vi "Abrir_central_todos_certificados.vi"() -> ()   [LabVIEW 2019]
uses:
  <vilib>/Utility/config.llb/Config Data RefNum.ctl
  <vilib>/Utility/config.llb/Write Key (Path).vi
  <vilib>/Utility/config.llb/NI_LVConfig.lvlib
panel:
  in  "Search Button":bool
  in  "barra_de_pesquisa":string
  in  "Editor Vinculos":bool
  in  "Stop Button":bool
  in  "Array":T1(array[cluster])
  out "Array Tags":string[](array[string])
  out "Section Names":string[](array[string])
  out "refnum out":T2
  out "error out":errorcluster
  # "Digite no campo de busca a TAG desejada:"
  # "Digite no campo de busca a TAG desejada:"
  # "SELECIONE A TAG A QUAL\nDESEJA ABRIR O PDF COM \nO CERTIFICADO DE CALIBRA敲O"
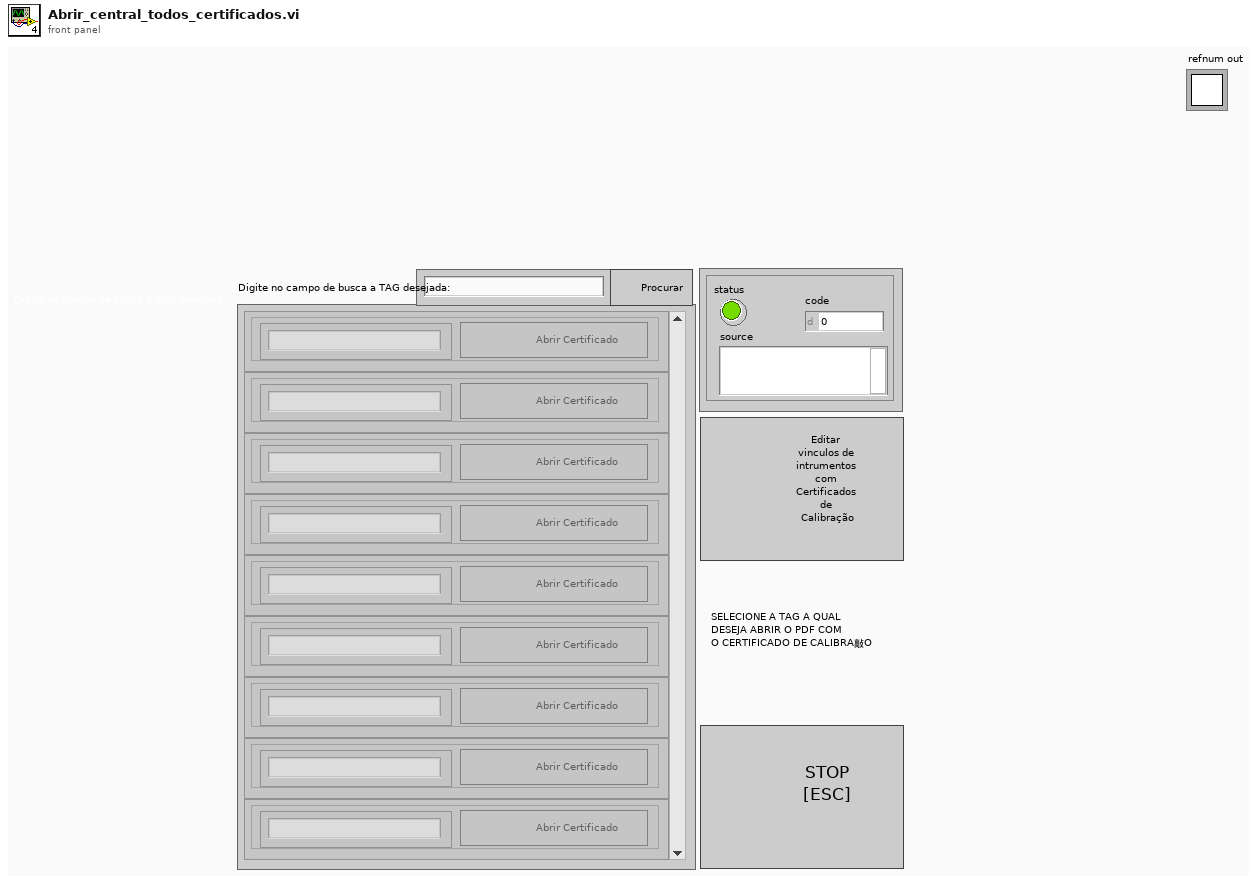
[diagram p1: front panel]
types:
  T1 = cluster{"TAG":string, "Abrir Certificado":bool}[]
  T2 = typedef "NI_LVConfig.lvlib/Config Data RefNum.ctl" = refnum<k1>
  T3 = enum8{"Enabled", "Disabled", "Disabled and Grayed Out"}
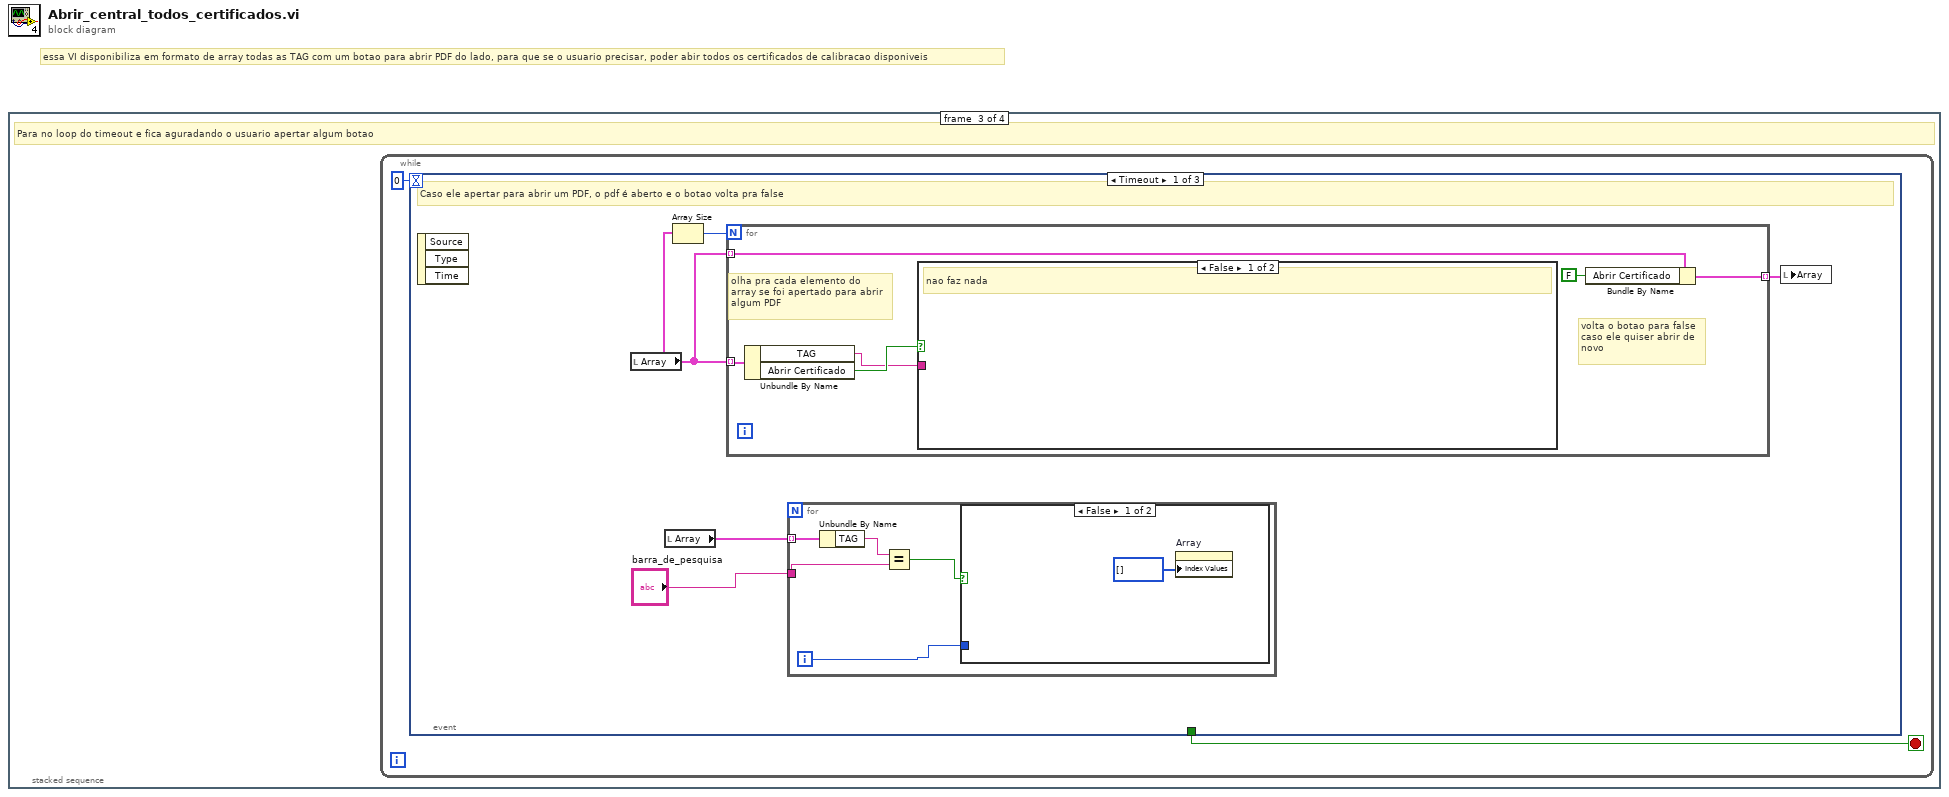
[diagram p0: block diagram]
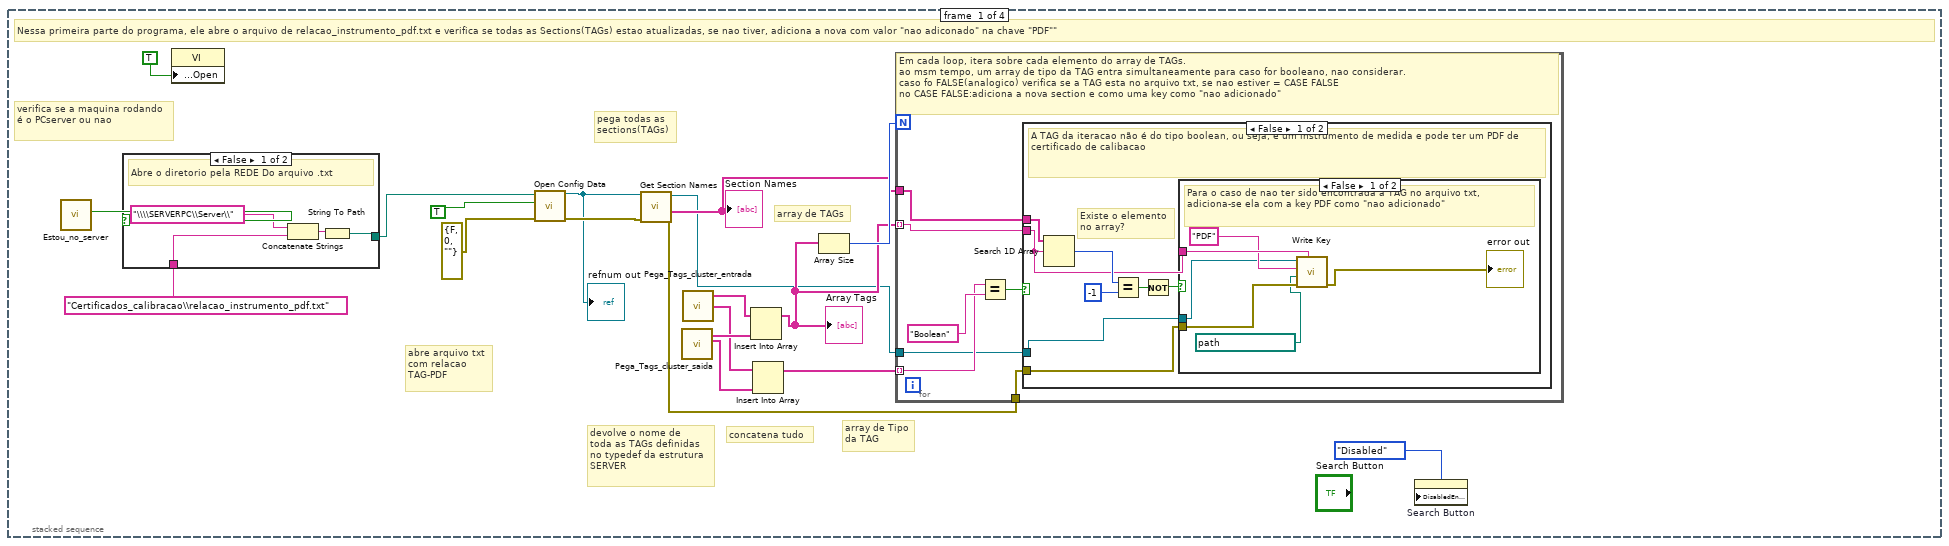
[diagram p2: hidden frame]
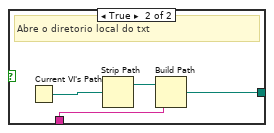
[diagram p3: hidden frame]
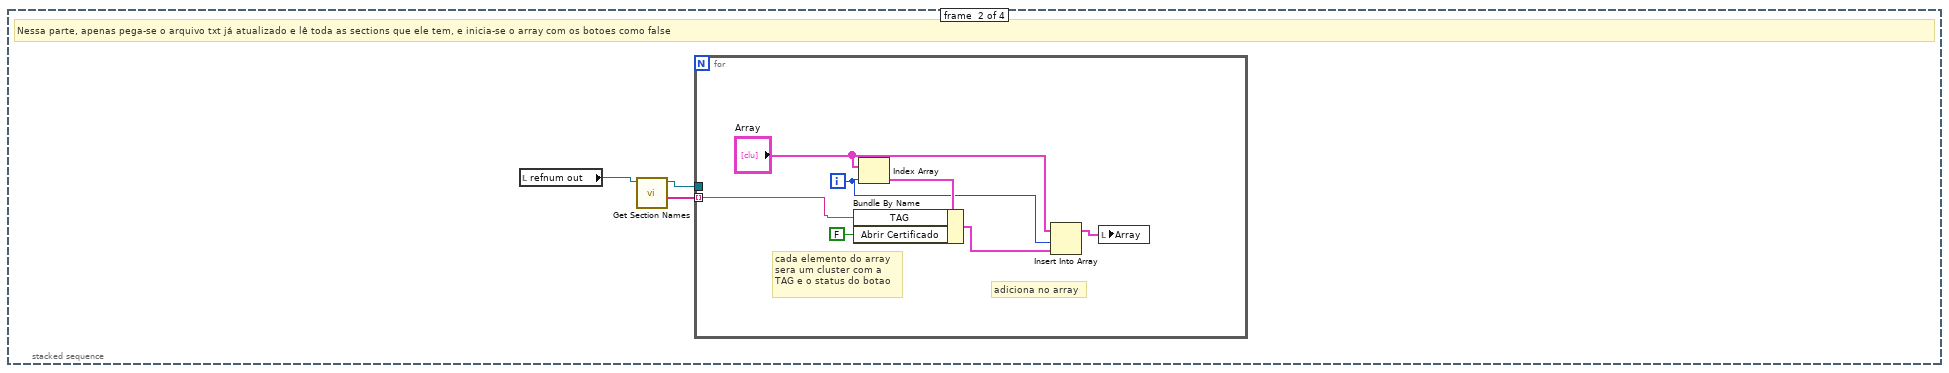
[diagram p6: hidden frame]
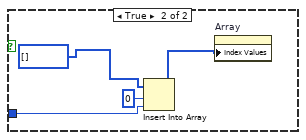
[diagram p7: hidden frame]
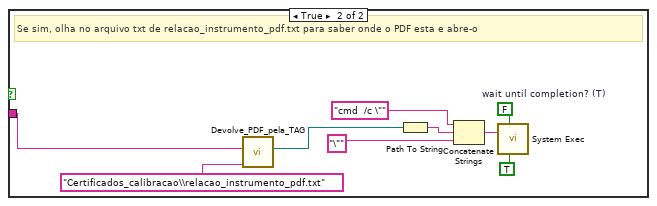
[diagram p8: hidden frame]
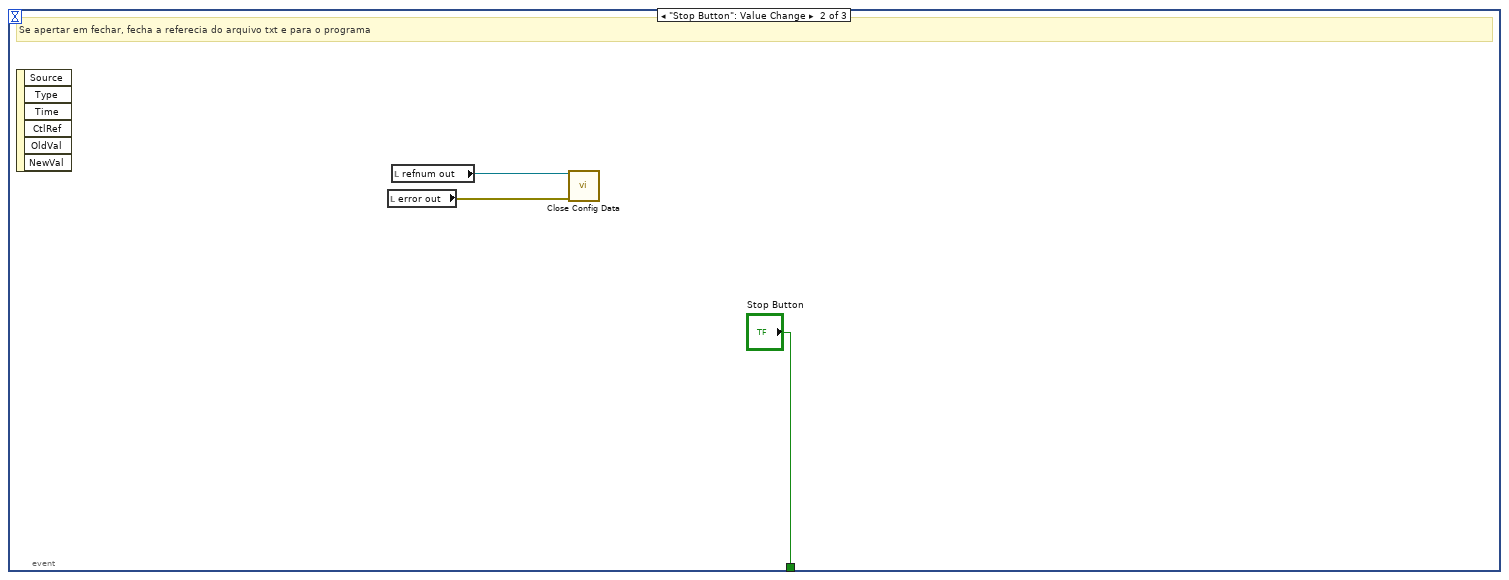
[diagram p9: hidden frame]
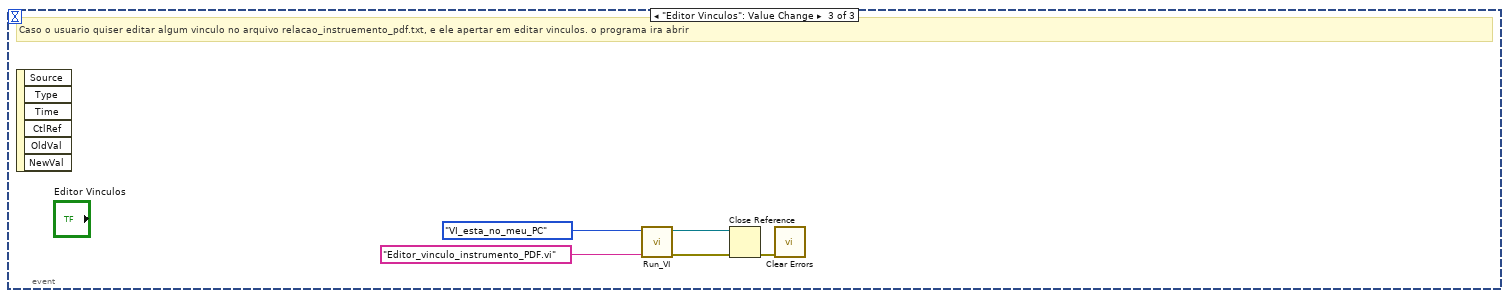
[diagram p10: hidden frame]
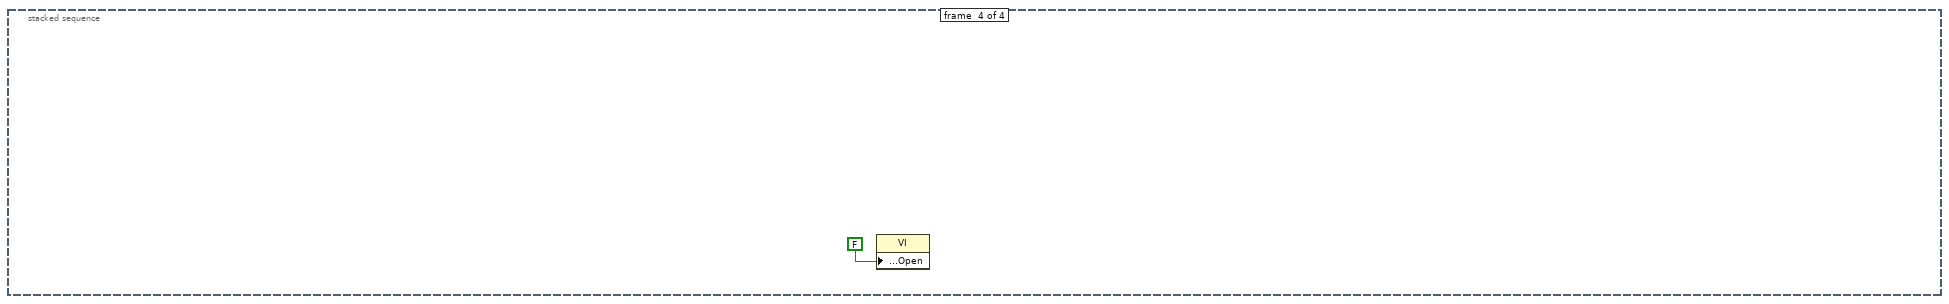
[diagram p11: hidden frame]
diagram:
  # "essa VI disponibiliza em formato de array todas as TAG com um botao para abrir PDF do lado, para que se o usuario precisar, poder abir todos os certificados de calibracao disponiveis"
  n1 = stacked-sequence {
    frame #0 {
      # "array de TAGs"
      # "array de Tipo\nda TAG"
      # "concatena tudo"
      # "devolve o nome de\ntoda as TAGs definidas\nno typedef da estrutura\nSERVER"
      # "pega todas as\nsections(TAGs)"
      # "abre arquivo txt\ncom relacao\nTAG-PDF"
      # "verifica se a maquina rodando é o PCserver ou nao"
      # "Nessa primeira parte do programa, ele abre o arquivo de relacao_instrumento_pdf.txt e verifica se todas as Sections(TAGs) estao atualizadas, se nao tiver, adiciona a nova com valor \"nao adiconado\" na chave \"PDF\"\""
      n2 = call "Estou_no_server.vi"() -> ("Estou no serve?"=w3:bool)  [unwired: 11 in]
      n3 = case shown="False" w3 {
        tunnel: [w21 w26] -> w2
        tunnel: "Certificados_calibracao\\relacao_instrumento_pdf.txt" ("name or relative path") -> [w22 w25]
        frame False {
          # "Abre o diretorio pela REDE Do arquivo .txt"
          n4 = Concatenate Strings("\\\\SERVERPC\\Server\\", w22) -> (w20:string)
          n5 = String To Path(string=w20) -> (path=w21:path)
        }
        frame True {
          # "Abre o diretorio local do txt"
          n6 = Current VI's Path() -> (path=w24:path)
          n7 = Strip Path(path=w24) -> (stripped path=w27:path)  [unwired: 1 out]
          n8 = Build Path(base path=w27, name or relative path=w25) -> (appended path=w26:path)
        }
      }
      n9 = property class="VI"("Front Panel.Open"=TRUE ("Front Panel Window:Open")) -> ()  [unwired: 2 in, 2 out]
      n10 = call <vilib>:"Open Config Data.vi"("error in (no error)"=errorcluster {"status"=FALSE, "code"=0, "source"=""}, "create file if necessary (T)"=TRUE, "configuration file path"=w2) -> ("error out"=w16:errorcluster, "refnum"=w15:T2)  [unwired: 6 in, 1 out]
      "refnum out" <- w15
      n11 = call <vilib>:"Get Section Names.vi"("error in (no error)"=w16, "refnum"=w15) -> ("error out"=w5:errorcluster, "section names"=w11:string[], "refnum out"=w6:T2)  [unwired: 7 in]
      "Section Names" <- w11
      n12 = call "Pega_Tags_cluster_saida.vi"() -> ("TipoTag"=w8:string[], "Array Tags"=w13:string[])  [unwired: 10 in]
      n13 = call "Pega_Tags_cluster_entrada.vi"() -> ("TipoVariavel"=w9:string[], "Array Tags"=w14:string[])  [unwired: 4 in]
      n14 = Insert Into Array(array=w14, new element=w13) -> (w10:string[])  [unwired: 1 in]
      "Array Tags" <- w10
      n15 = Insert Into Array(array=w9, new element=w8) -> (w7:string[])  [unwired: 1 in]
      n16 = Array Size(array=w10) -> (size(s)=w12:i32)
      n17 = for {
        N: w12 -> [_]
        tunnel: w10 -> [w31] mode=indexing
        tunnel: w11 -> [w30]
        tunnel: w7 -> [w33] mode=indexing
        tunnel: w6 -> [w29]
        tunnel: w5 -> [w28]
        # "Em cada loop, itera sobre cada elemento do array de TAGs.\nao msm tempo, um array de tipo da TAG entra simultaneamente para caso for booleano, nao considerar.\ncaso fo FALSE(analogico) verifica se a TAG esta no arquivo txt, se nao estiver = CASE FALSE\nno CASE FALSE:adiciona a nova section e como uma key como \"nao adicionado\""
        n18 = Equal?(x=w33, y="Boolean") -> (x = y?=w32:bool)
        n19 = case shown="False" w32 {
          tunnel: w31 -> [w37 _]
          tunnel: w30 -> [w40 _]
          tunnel: w29 -> [w36 _]
          tunnel: w28 -> [w35 _]
          frame False {
            # "Existe o elemento\nno array?"
            # "A TAG da iteracao não é do tipo boolean, ou seja, é um instrumento de medida e pode ter um PDF de certificado de calibacao"
            n20 = Search 1D Array(1D array=w40, element=w37) -> (index of element=w39:i32)  [unwired: 1 in]
            n21 = Equal?(x=w39, y=-1) -> (x = y?=w42:bool)
            n22 = Not(x=w42) -> (.not. x?=w38:bool)
            n23 = case shown="False" w38 {
              tunnel: w37 -> [w48 _]
              tunnel: w36 -> [w46 _]
              tunnel: w35 -> [w45 _]
              frame False {
                # "Para o caso de nao ter sido encontrada a TAG no arquivo txt,\nadiciona-se ela com a key PDF como \"nao adicionado\""
                n24 = call-poly <vilib>:"Write Key.vi"("section"=w48, "error in (no error)"=w45, "value"=path "Não Adicionado", "key"="PDF", "refnum"=w46) -> ("error out"=→"error out":errorcluster)  [unwired: 4 in, 2 out]
              }
              frame True {
              }
            }
          }
          frame True {
            # "a TAG analisada é uma booleana"
          }
        }
      }
      n25 = property on="Search Button" class="Bool"("DisabledEnum"=T3."Disabled" ("Disabled")) -> ()  [unwired: 2 in, 2 out]
    }
    frame #1 {
      # "Nessa parte, apenas pega-se o arquivo txt já atualizado e lê toda as sections que ele tem, e inicia-se o array com os botoes como false"
      n26 = local read "refnum out"() -> (w51:T2)
      n27 = call <vilib>:"Get Section Names.vi"("refnum"=w51) -> ("section names"=w50:string[], "refnum out"=w49:T2)  [unwired: 8 in, 1 out]
      n28 = for {
        tunnel: w50 -> [w55] mode=indexing
        tunnel: w49 -> [_]
        i -> [w56]
        # "adiciona no array"
        # "cada elemento do array\nsera um cluster com a \nTAG e o status do botao"
        n29 = Index Array(array="Array", index=w56) -> (element=w58:cluster{"TAG":string, "Abrir Certificado":bool})
        n30 = Bundle By Name(cluster=w58, "TAG"=w55, "Abrir Certificado"=FALSE) -> (w57:cluster{"TAG":string, "Abrir Certificado":bool})
        n31 = Insert Into Array(array="Array", index=w56, new element=w57) -> (w53:T1)
        n32 = local write "Array"(w53) -> ()
      }
    }
    frame #2 {
      # "Para no loop do timeout e fica aguradando o usuario apertar algum botao"
      n33 = while {
        stop <- w60 stop-if-true
        n34 = event shown="[0] Timeout" {
          selector: _ -> [_ _ _]
          dyn-events: _ -> [_ _ _]
          timeout: 0 -> [_ _ _]
          tunnel: [_ "Stop Button" _] -> w60
          event Timeout {
            # "Caso ele apertar para abrir um PDF, o pdf é aberto e o botao volta pra false"
            n35 = event-data() -> ()  [unwired: 1 in, 3 out]
            n36 = local read "Array"() -> (w65:T1)
            n37 = local read "Array"() -> (w62:T1)
            n38 = Array Size(array=w65) -> (size(s)=w64:i32)
            n39 = for {
              N: w64 -> [_]
              tunnel: w65 -> [w81] mode=indexing
              tunnel: w65 -> [w78] mode=indexing
              tunnel: [w77] -> w63 mode=indexing
              # "volta o botao para false\ncaso ele quiser abrir de \nnovo"
              # "olha pra cada elemento do\narray se foi apertado para abrir\nalgum PDF"
              n40 = Unbundle By Name(w81) -> ("TAG"=w79:string, "Abrir Certificado"=w80:bool)
              n41 = case shown="False" w80 {
                tunnel: w79 -> [_ w90]
                frame False {
                  # "nao faz nada"
                }
                frame True {
                  w88 = FALSE  # wait until completion? (T)
                  # "Se sim, olha no arquivo txt de relacao_instrumento_pdf.txt para saber onde o PDF esta e abre-o"
                  n42 = call "Devolve_PDF_pela_TAG.vi"("caminho_relacao_instrumento_PDF_txt"="Certificados_calibracao\\relacao_instrumento_pdf.txt" ("name or relative path"), "TAG"=w90) -> ("path"=w89:path)  [unwired: 5 in, 2 out]
                  n43 = Path To String(path=w89) -> (string=w84:string)
                  n44 = Concatenate Strings("cmd  /c \"", w84, "\"") -> (w86:string)
                  n45 = call <vilib>:"System Exec.vi"("run minimized? (F)"=TRUE, "wait until completion? (T)"=w88, "command line"=w86) -> ()  [unwired: 5 in, 4 out]
                }
              }
              n46 = Bundle By Name(cluster=w78, "Abrir Certificado"=FALSE) -> (w77:cluster{"TAG":string, "Abrir Certificado":bool})
            }
            n47 = for {
              tunnel: w62 -> [w70] mode=indexing
              tunnel: "barra_de_pesquisa" -> [w68]
              i -> [w67]
              n48 = Unbundle By Name(w70) -> ("TAG"=w69:string)
              n49 = Equal?(x=w69, y=w68) -> (x = y?=w66:bool)
              n50 = case shown="False" w66 {
                tunnel: w67 -> [_ w74]
                frame False {
                  n51 = property on="Array" class="Arr"("Index Values"=u32[] []) -> ()  [unwired: 2 in, 2 out]
                }
                frame True {
                  n52 = Insert Into Array(array=u32[] [] ("Index Values"), index=0, new element=w74) -> (w72:u32[])
                  n53 = property on="Array" class="Arr"("Index Values"=w72) -> ()  [unwired: 2 in, 2 out]
                }
              }
            }
            n54 = local write "Array"(w63) -> ()
          }
          event "Stop Button": Value Change {
            # "Se apertar em fechar, fecha a referecia do arquivo txt e para o programa"
            n55 = event-data() -> ()  [unwired: 1 in, 6 out]
            n56 = local read "error out"() -> (w91:errorcluster)
            n57 = local read "refnum out"() -> (w92:T2)
            n58 = call <vilib>:"Close Config Data.vi"("error in (no error)"=w91, "refnum"=w92) -> ()  [unwired: 8 in, 2 out]
          }
          event "Editor Vinculos": Value Change {
            # "Caso o usuario quiser editar algum vinculo no arquivo relacao_instruemento_pdf.txt, e ele apertar em editar vinculos. o programa ira abrir"
            n59 = event-data() -> ()  [unwired: 1 in, 6 out]
            n60 = call "Run_VI.vi"("Nome.vi"="Editor_vinculo_instrumento_PDF.vi", "Origem_VI"=enum16{"VI_esta_no_meu_PC", "VI_esta_na_rede"}."VI_esta_no_meu_PC") -> ("error out"=w97:errorcluster, "reference out"=w98:refnum<vi>)  [unwired: 8 in]
            n61 = Close Reference(reference=w98, error in (no error)=w97) -> (error out=w96:errorcluster)
            n62 = call <vilib>:"Clear Errors.vi"("error in (no error)"=w96) -> ()  [unwired: 5 in, 2 out]
          }
        }
      }
    }
    frame #3 {
      n63 = property class="VI"("Front Panel.Open"=FALSE ("Front Panel Window:Open")) -> ()  [unwired: 2 in, 2 out]
    }
  }
